vi "create incident - warning.vi"(9 "warning description":string="unhandled message :", 11 "RT Queues":T1) -> (3 "RT Queues out":T1)   [LabVIEW 2018]
uses:
  Type Defs/Queues cluster.ctl
  ICL-LabVIEW_General/Message Scheduler/message scheduler.lvclass
  Type Defs/warning incident cluster.ctl
  Queue VIs/En-queue RT comms element.vi
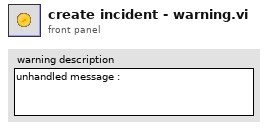
[diagram p1: front panel]
types:
  T1 = typedef "Queues cluster.ctl" = cluster{"RT Message":refnum<queue>, "RT Comms":refnum<queue>, "RT Data":refnum<queue>, "RT FIFO":refnum<queue>, "message scheduler":refnum<class "message scheduler.lvclass">}
  T2 = typedef "warning incident cluster.ctl" = cluster{"warning description":string, "call chain":string[]}
  T3 = cluster{"seconds since 1Jan1904":timestamp, "type":string, "Variant":variant}
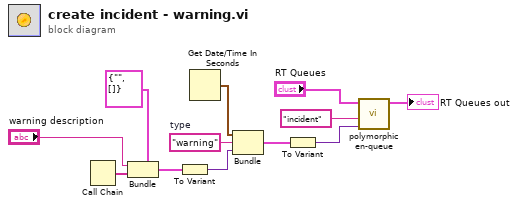
[diagram p0: block diagram]
diagram:
  w9 = "warning"  # type
  n1 = Call Chain() -> (call chain=w12:string[])
  n2 = Bundle(cluster=T2 {"warning description"="", "call chain"=[]}, "warning description"="warning description", "call chain"=w12) -> (w8:T2)
  n3 = To Variant(anything=w8) -> (Variant=w7:variant)
  n4 = Get Date/Time In Seconds() -> (seconds since 1Jan1904=w4:timestamp)
  n5 = Bundle("seconds since 1Jan1904"=w4, "type"=w9, "Variant"=w7) -> (w6:T3)  [unwired: 1 in]
  n6 = To Variant(anything=w6) -> (Variant=w5:variant)
  n7 = call-poly "polymorphic en-queue.vi"("Data"=w5, "Message"="incident", "RT Queues"="RT Queues") -> ("RT Queues out"=→"RT Queues out":T1)  [unwired: 8 in]
